vi "4Pi Dual DM - Mode Scan Engine.vi"() -> ()   [LabVIEW 2016]
uses:
  4Pi Dual DM - Controls/4Pi Dual DM - Mode Scan - Gaussian Initial Guesses.ctl
  4Pi Dual DM - Controls/4Pi Dual DM - Mode Scan - Metric Fit Type.ctl
  4Pi Dual DM - Controls/4Pi Dual DM - Mode Scan - Scan Settings.ctl
  4Pi Dual DM - Controls/4Pi Dual DM - Mode Scan - Metric.ctl
  4Pi Dual DM - Controls/4Pi Dual DM - Mode Scan - Threshold Mean Limits.ctl
  4Pi Dual DM - Controls/4Pi Dual DM - Mode Scan - Image Type.ctl
  4Pi Dual DM - Controls/4Pi Dual DM - Mode Scan - Blink Scan Settings.ctl
  4Pi Dual DM - Controls/4Pi Dual DM - Mode Scan - Blink Analysis Type.ctl
  <vilib>/vision/Image Controls.llb/IMAQ Image.ctl
  Hardware Configuration/Hardware Configuration Controls/Device Type.ctl
  Hardware Configuration/Hardware Configuration Controls/Device Function.ctl
  <vilib>/Utility/miscctls.llb/LVPointTypeDef.ctl
  4Pi Dual DM - Controls/4Pi Dual DM - Mode Scan - Last Used Data Type.ctl
  4Pi Dual DM - Controls/4Pi Dual DM - Mode Scan - Notifier Type.ctl
  4Pi Dual DM - Controls/4Pi Dual DM - Mode Scan - Scan Actions.ctl
  4Pi Dual DM - Controls/4Pi Dual DM - Standard Action.ctl
  4Pi Dual DM - Controls/4Pi Dual DM - Standard Counter Action.ctl
  <vilib>/Analysis/6fits.llb/Curve Fitting Criteria.ctl
  <vilib>/Analysis/baseanly.llb/Mean (DBL).vi
  <vilib>/Analysis/NI_AALBase.lvlib
  <vilib>/Analysis/NI_AALPro.lvlib
  <vilib>/gmath/NI_Gmath.lvlib
  <resource>/objmgr/IMAQImage.rc
panel:
  in  "Current Mode":i32(ring) items=["1", "2", "3", "4", "5", "6", "7", "8", "9", "10", "11", "12", "13", "14", "15", "16", "17", "18", "19", "20", "21", "22", "23", "24", "25", "26", "27", "28", "29", "30", "31", "32", "33", "34", "35", "36", "37", "38", "39", "40", "41", "42", "43", "44", "45", "46", "47", "48", "49", "50", "51", "52", "53", "54", "55", "56", "57", "58", "59", "60", "61", "62", "63", "64", "65", "66", "67", "68", "69", "70", "71", "72", "73", "74", "75", "76", "77", "78", "79", "80", "81", "82", "83", "84", "85", "86", "87", "88", "89", "90", "91", "92", "93", "94", "95", "96", "97", "98", "99", "100", "101", "102", "103", "104", "105", "106", "107", "108", "109", "110", "111", "112", "113", "114", "115", "116", "117", "118", "119", "120", "121", "122", "123", "124", "125", "126", "127", "128", "129", "130", "131", "132", "133", "134", "135", "136", "137", "138", "139", "140"]
  in  "Scan Mode":bool
  in  "Scan Next Mode":bool
  in  "Auto Scan Modes":bool
  in  "Calling VI Ref":refnum<vi>
  in  "Main Tab":enum32{"Scan Modes", "Settings"}(tab)
  in  "Blink Scan Settings":T1={"Blink Analysis Type"=1, "Blink ROI Box Width"=0, "Blink Threshold"=0.0} {"Blink Analysis Type" items=["Mean Intensity", "2D Fit Intensity"]}
  in  "Fit Data":bool
  in  "Apply":bool
  in  "Get Image":bool
  in  "Image Type":T3 items=["Full Image", "ROI", "Blinks"]
  in  "Fit Type":T4 items=["Guassian", "Quadratic"]
  in  "Gaussian Initial Guesses":T5={"Amplitude"=2500.0, "Center Position"=0.0, "Width (Sigma)"=200.0, "Offset"=500.0, "User Guesses"=TRUE}
  in  "DM Scan Settings":T6={"Frame Delay"=1, "Frame Accumulations"=2, "Number of Steps"=8, "Step Size (nm)"=80}
  in  "Metric":T7=1 items=["Max Intensity", "No Zero Mean", "Threshold Mean", "Mean"]
  in  "Image Selection":i32(ring) items=["Quad 01", "Quad 02", "Quad 03", "Quad 04"]
  in  "Threshold Mean Limits":T8={"Upper Limit"=10000.0, "Lower Limit"=0.0}
  out "Metric":cluster{dbl[], dbl[]}[](graph)
  out "Image":u16[][](graph)
  in  "Exit":bool
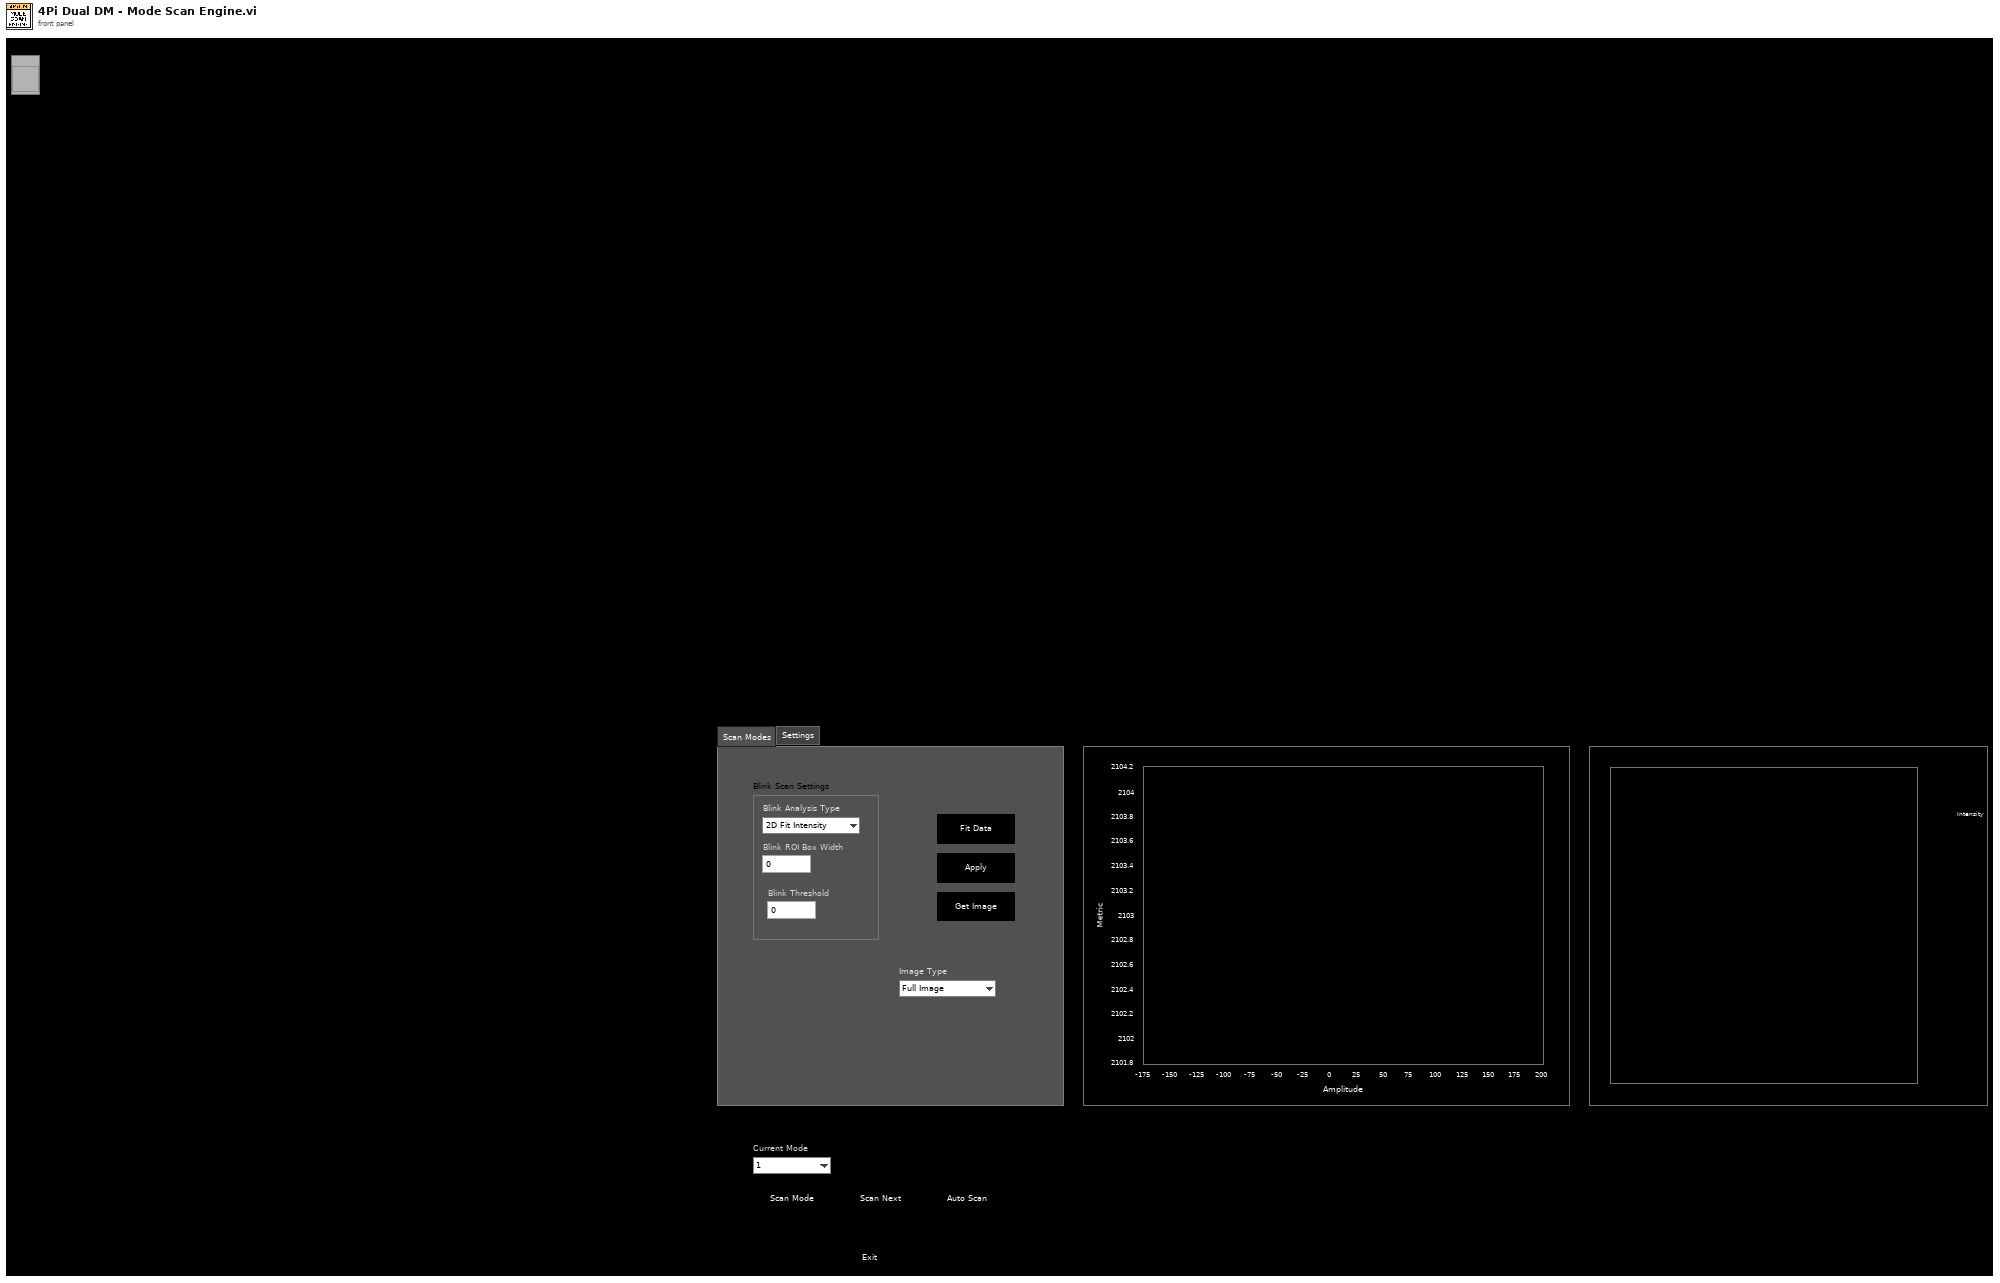
[diagram p1: front panel]
types:
  T1 = typedef "4Pi Dual DM - Mode Scan - Blink Scan Settings.ctl" = cluster{"Blink Analysis Type":T2, "Blink ROI Box Width":u8, "Blink Threshold":dbl}
  T2 = typedef "4Pi Dual DM - Mode Scan - Blink Analysis Type.ctl" = u16
  T3 = typedef "4Pi Dual DM - Mode Scan - Image Type.ctl" = u16
  T4 = typedef "4Pi Dual DM - Mode Scan - Metric Fit Type.ctl" = u16
  T5 = typedef "4Pi Dual DM - Mode Scan - Gaussian Initial Guesses.ctl" = cluster{"Amplitude":dbl, "Center Position":dbl, "Width (Sigma)":dbl, "Offset":dbl, "User Guesses":bool}
  T6 = typedef "4Pi Dual DM - Mode Scan - Scan Settings.ctl" = cluster{"Frame Delay":u32, "Frame Accumulations":u16, "Number of Steps":u16, "Step Size (nm)":u16}
  T7 = typedef "4Pi Dual DM - Mode Scan - Metric.ctl" = u16
  T8 = typedef "4Pi Dual DM - Mode Scan - Threshold Mean Limits.ctl" = cluster{"Upper Limit":dbl, "Lower Limit":dbl}
  T9 = typedef "4Pi Dual DM - Mode Scan - Scan Actions.ctl" = enum16{"Scan Mode", "Fit Data", "Scan Next Mode", "Update Mode Amount", "Get Image", "Compute Metric", "Update Counter", "Apply Correction", "Exit", "Quit"}
  T10 = typedef "4Pi Dual DM - Mode Scan - Notifier Type.ctl" = cluster{"Action":T9, "Image Ref":T11, "Image Type":T3, "Fit Type":T4, "Metric":T7, "Scan Running?":bool, "DM Scan Settings":T6, "Threshold Mean Limits":T8, "Gaussian Initial Guesses":T5, "Blink Scan Settings":T1}
  T11 = typedef "IMAQ Image.ctl" = refnum<image>
  T12 = typedef "4Pi Dual DM - Mode Scan - Last Used Data Type.ctl" = cluster{"Image Ref Index":i32, "Image Type":T3, "Fit Type":T4, "Metric":T7, "DM Scan Settings":T6, "Threshold Mean Limits":T8, "Gaussian Initial Guesses":T5, "Blink Scan Settings":T1}
  T13 = enum16{"Always On", "Always Off", "Off While Running"}
  T14 = typedef "LVPointTypeDef.ctl" = cluster{"Horizontal":i16, "Vertical":i16}
  T15 = typedef "Device Function.ctl" = enum16{"Primary", "Secondary", "Overview", "Wide Field Drift Correction", "642 nm Excitation", "560 nm Excitation", "546 nm Excitation", "488 nm Excitation", "405 nm Excitation", "Objective Drift Correction", "Objective XY", "Objective Z", "Sample XY", "Sample Coarse Z", "Sample Z", "4Pi Lower", "4Pi Upper", "Adj Cavity", "Line Scanning"}
  T16 = typedef "Device Type.ctl" = enum16{"AOTF", "Camera", "Deformable Mirror", "Laser", "Shutter", "Stage", "Waveform"}
  T17 = typedef "LVRectTypeDef.ctl" = cluster{"Left":i16, "Top":i16, "Right":i16, "Bottom":i16}
  T18 = typedef "LVBoundsTypeDef.ctl" = cluster{"Width":u32, "Height":u32}
  T19 = typedef "4Pi Dual DM - Standard Action.ctl" = enum16{"Read", "Write"}
  T20 = typedef "4Pi Dual DM - Standard Counter Action.ctl" = enum16{"Initialize", "Update Count", "Get Count"}
  T21 = cluster{"initial amplitude":dbl, "initial center":dbl, "initial standard deviation":dbl, "offset":dbl}
  T22 = cluster{"amp min":dbl, "amp max":dbl, "center min":dbl, "center max":dbl, "deviation min":dbl, "deviation max":dbl, "offset min":dbl, "offset max":dbl}
  T23 = enum16{"Linear", "Polynomial", "Exponential", "Power"}
  T24 = enum8{"Enabled", "Disabled", "Disabled and Grayed Out"}
  T25 = typedef "4Pi Dual DM - Mirror Modes DUAL.ctl" = cluster{"Mode":string, "Amplitude":dbl}[][]
  T26 = cluster{"Amplitude Out":dbl[], "Metric Out":dbl[]}
  T27 = cluster{"initial amplitude":dbl, "Numeric":dbl, "initial standard deviation":dbl, "offset":dbl}
  T28 = typedef "NI_AALPro.lvlib/Curve Fitting Criteria.ctl" = u16
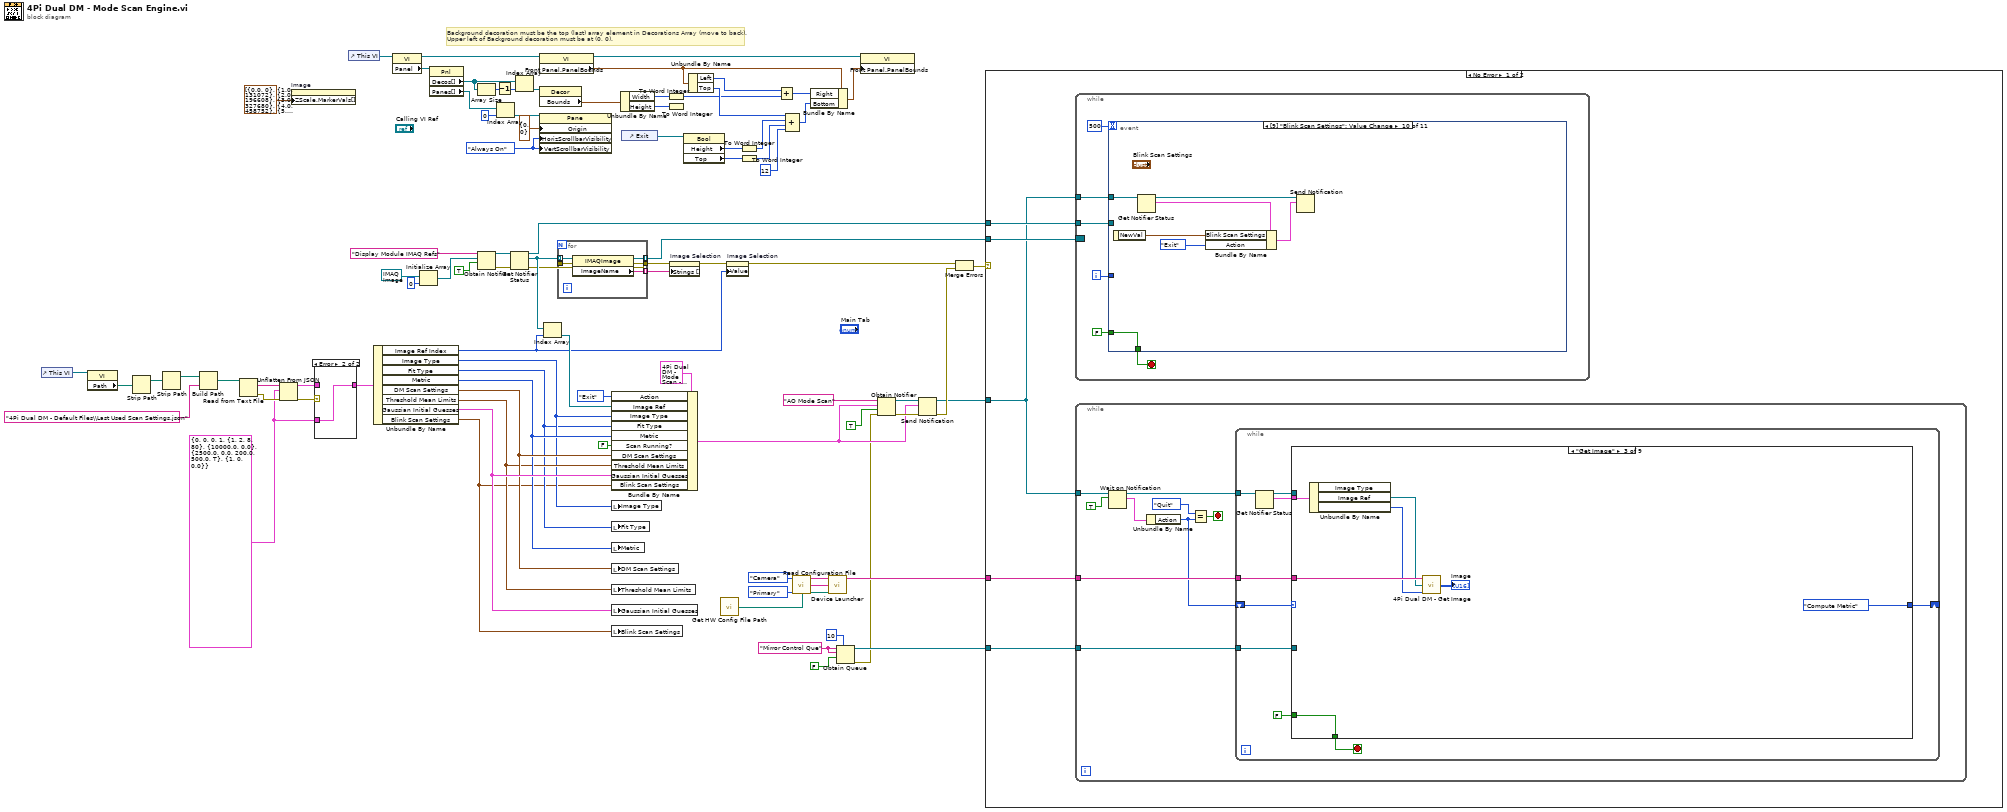
[diagram p0: block diagram]
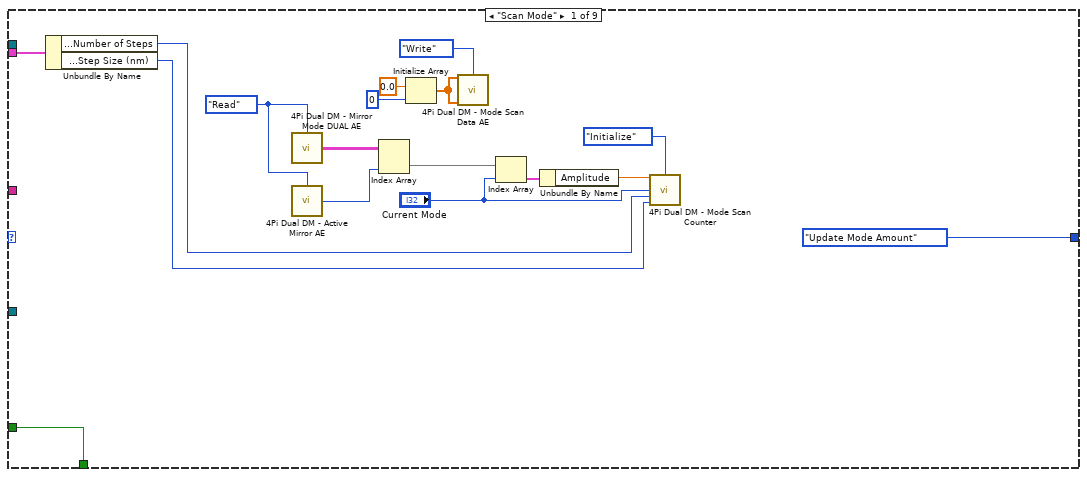
[diagram p2: hidden frame]
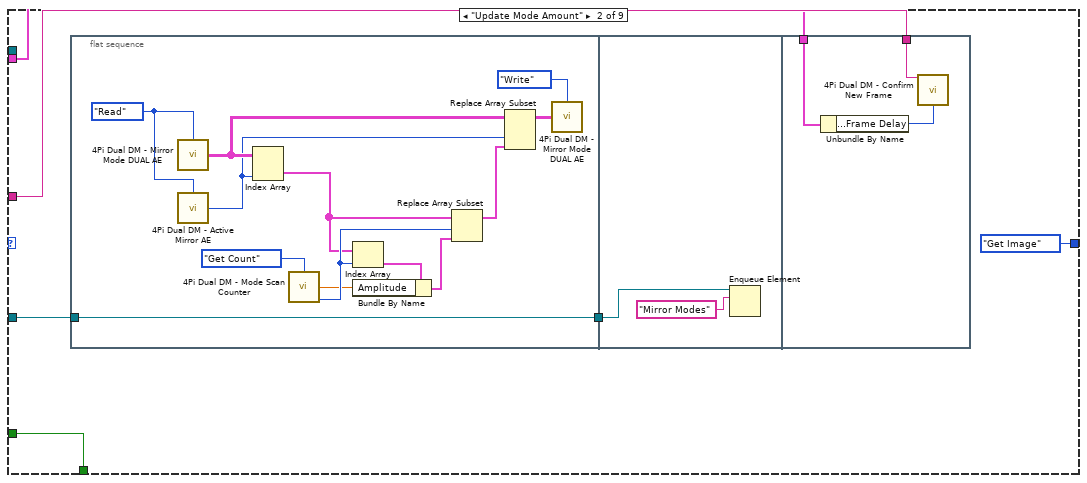
[diagram p3: hidden frame]
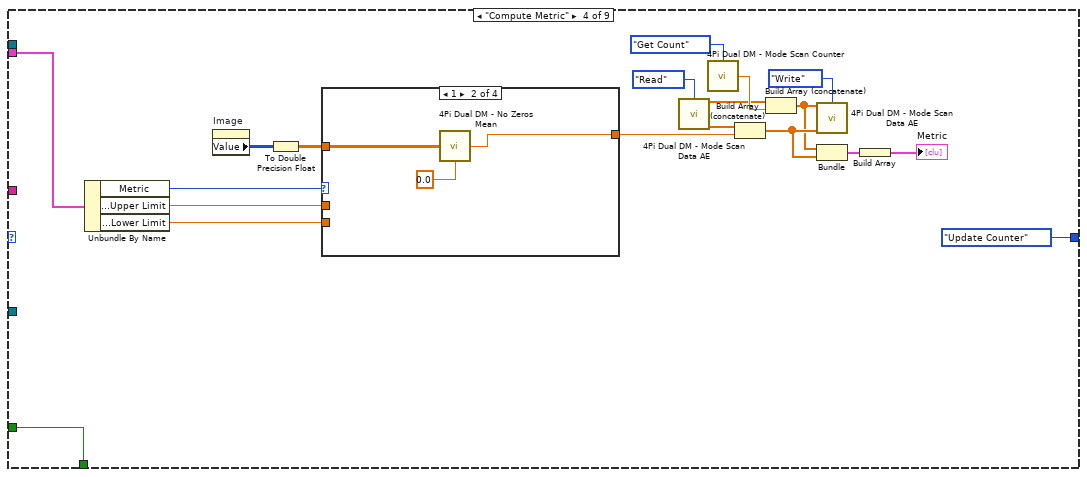
[diagram p4: hidden frame]
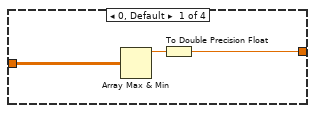
[diagram p5: hidden frame]
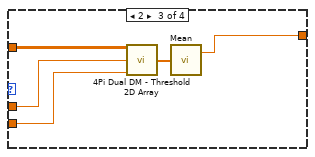
[diagram p6: hidden frame]
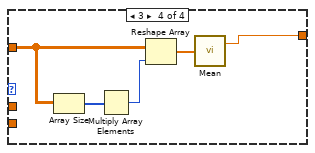
[diagram p7: hidden frame]
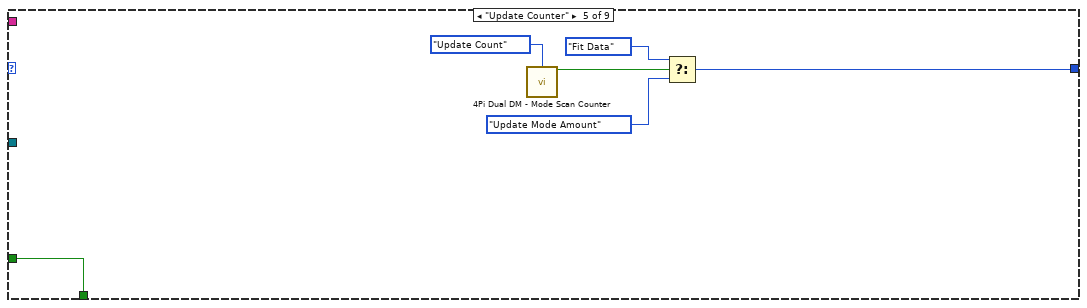
[diagram p8: hidden frame]
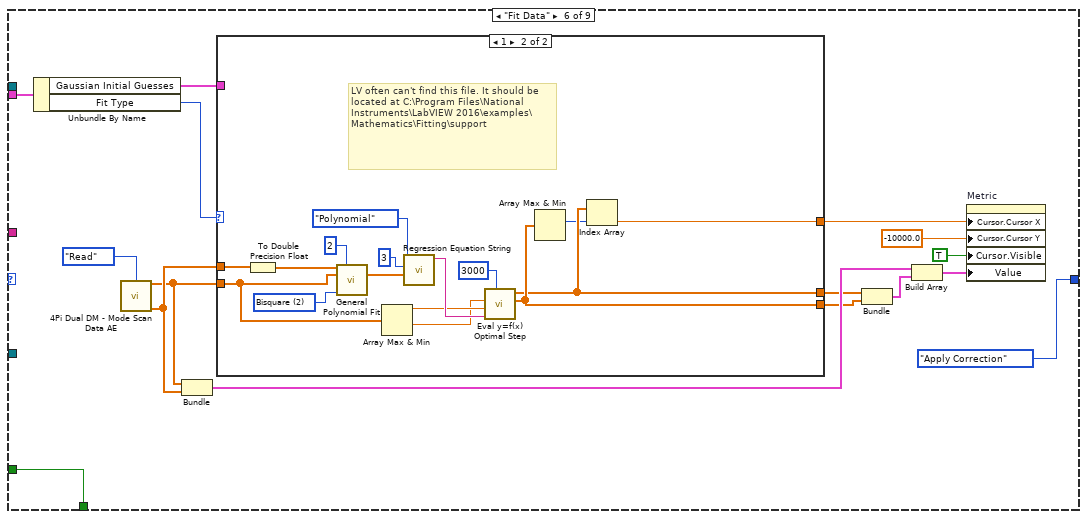
[diagram p9: hidden frame]
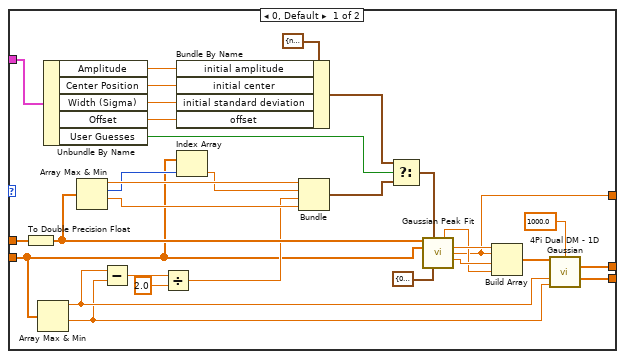
[diagram p10: hidden frame]
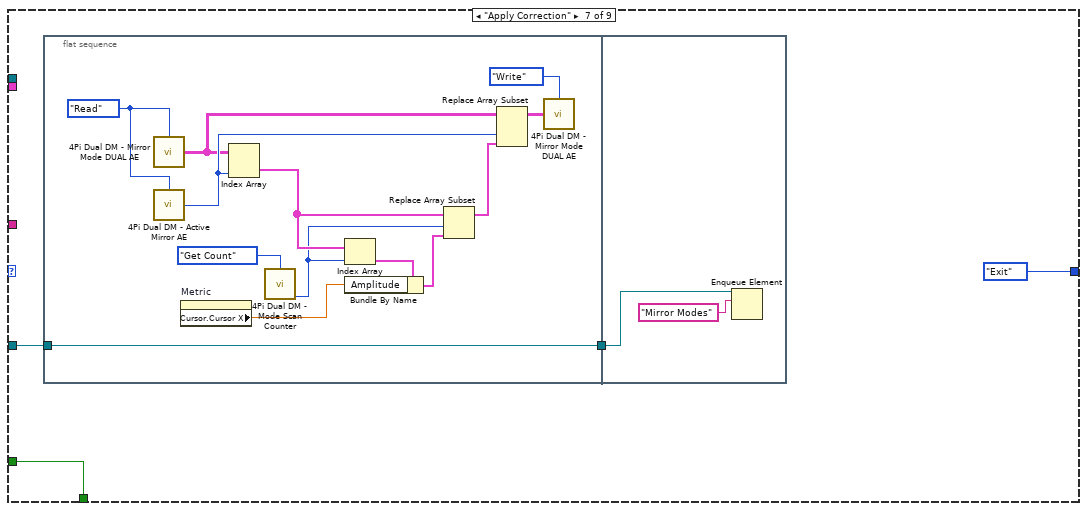
[diagram p11: hidden frame]
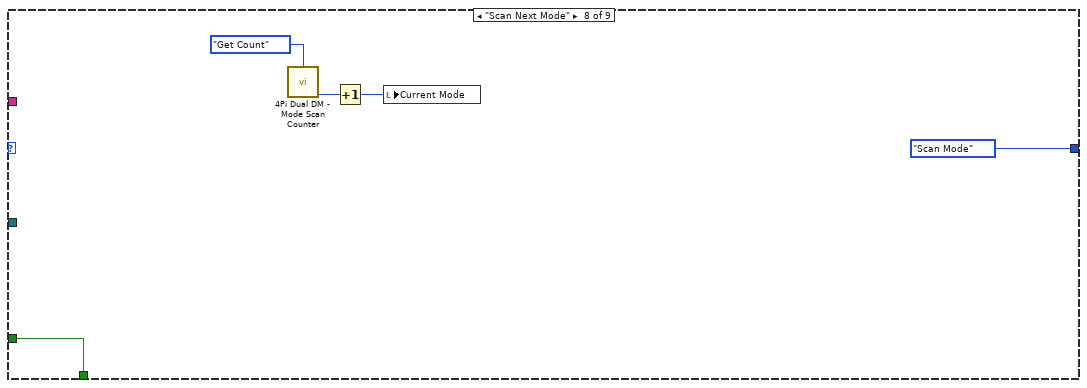
[diagram p12: hidden frame]
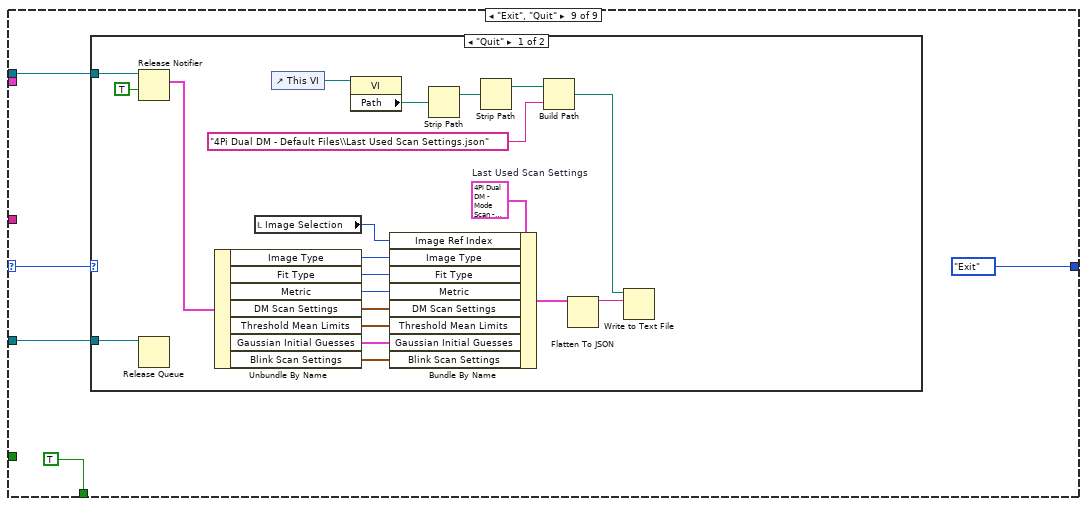
[diagram p13: hidden frame]
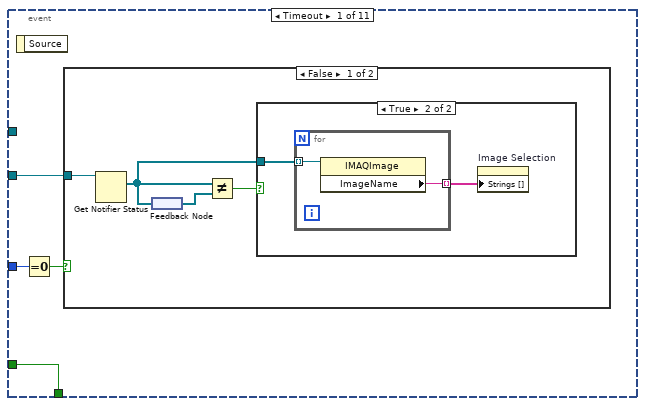
[diagram p15: hidden frame]
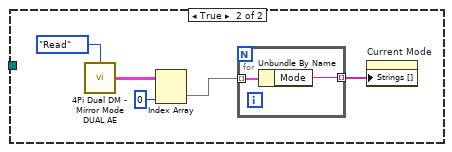
[diagram p17: hidden frame]
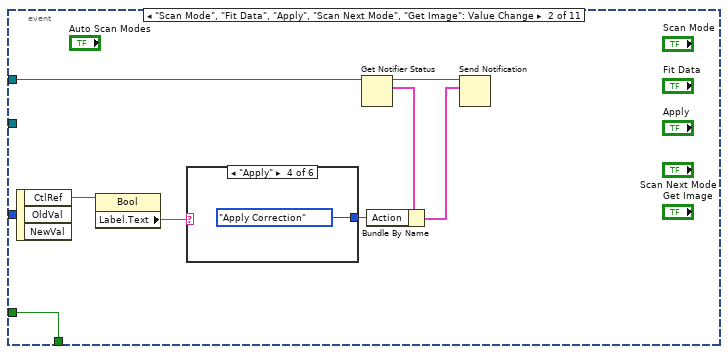
[diagram p18: hidden frame]
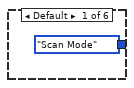
[diagram p19: hidden frame]
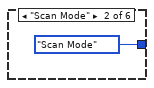
[diagram p20: hidden frame]
diagram:
  w24 = T12 {"Image Ref Index"=0, "Image Type"=0, "Fit Type"=0, "Metric"=1, "DM Scan Settings"={"Frame Delay"=1, "Frame Accumulations"=2, "Number of Steps"=8, "Step Size (nm)"=80}, "Threshold Mean Limits"={"Upper Limit"=10000.0, "Lower Limit"=0.0}, "Gaussian Initial Guesses"={"Amplitude"=2500.0, "Center Position"=0.0, "Width (Sigma)"=200.0, "Offset"=500.0, "User Guesses"=TRUE}, "Blink Scan Settings"={"Blink Analysis Type"=1, "Blink ROI Box Width"=0, "Blink Threshold"=0.0}} ("Mode Scan Notifier Type")
  w55 = T13."Always On" ("Vertical Scrollbar Visibility")
  w89 = "Mirror Control Que" ("name (unnamed)")
  # "Background decoration must be the top (last) array element in Decorations Array (move to back).\nUpper left of Background decoration must be at (0, 0)."
  n1 = control-ref of="This VI"() -> (w37:refnum<vi>)
  n2 = property class="VI"(reference=w37) -> ("Path"=w36:path)  [unwired: 1 in, 2 out]
  n3 = Strip Path(path=w36) -> (stripped path=w35:path)  [unwired: 1 out]
  n4 = Strip Path(path=w35) -> (stripped path=w34:path)  [unwired: 1 out]
  n5 = Build Path(base path=w34, name or relative path="4Pi Dual DM - Default Files\\Last Used Scan Settings.json") -> (appended path=w31:path)
  n6 = Read from Text File(file (use dialog)=w31) -> (text=w32:string, error out=w30:errorcluster)  [unwired: 3 in, 2 out]
  n7 = Unflatten From JSON(JSON string=w32, type and defaults=w24, error in (no error)=w30) -> (value=w23:T12, error out=w29:errorcluster)  [unwired: 4 in]
  n8 = property on="Image" class="IntGraph (strict)"("ZScale.MarkerVals[]"=cluster{dbl, u32}[] [{0.0, 0}, {1.0, 131072}, {2.0, 196608}, {3.0, 327680}, {4.0, 458752}, {5.0, 589824}, {6.0, 720896}, {7.0, 851971}, {8.0, 983043}, {9.0, 1114115}, {10.0, 1245187}, {11.0, 1376259}, {12.0, 1507331}, {13.0, 1638403}, {14.0, 1769475}, {15.0, 1769479}, {16.0, 2031623}, {17.0, 2162695}, {18.0, 2293767}, {19.0, 2424839}, {20.0, 2555911}, {21.0, 2686983}, {22.0, 2818055}, {23.0, 2949127}, {24.0, 3080203}, {25.0, 3211275}, {26.0, 3342347}, {27.0, 3473419}, {28.0, 3604491}, {29.0, 3735563}, {30.0, 3866635}, {31.0, 3867403}, {32.0, 4129547}, {33.0, 4260619}, {34.0, 4391691}, {35.0, 4522763}, {36.0, 4653839}, {37.0, 4784911}, {38.0, 4915983}, {39.0, 5178127}, {40.0, 5309199}, {41.0, 5440271}, {42.0, 5571343}, {43.0, 5702415}, {44.0, 5703439}, {45.0, 5965583}, {46.0, 6096655}, {47.0, 6227727}, {48.0, 6358799}, {49.0, 6489871}, {50.0, 6620943}, {51.0, 6752015}, {52.0, 6883087}, {53.0, 7015183}, {54.0, 7146255}, {55.0, 7277327}, {56.0, 7408399}, {57.0, 7539471}, {58.0, 7670543}, {59.0, 7801615}, {60.0, 8063759}, {61.0, 8194831}, {62.0, 8326927}, {63.0, 8457999}, {64.0, 8589075}, {65.0, 8720147}, {66.0, 8851219}, {67.0, 8982291}, {68.0, 9113363}, {69.0, 9114387}, {70.0, 9376531}, {71.0, 9507603}, {72.0, 9638675}, {73.0, 9769747}, {74.0, 9901843}, {75.0, 10032915}, {76.0, 10163987}, {77.0, 10229523}, {78.0, 10295059}, {79.0, 10427155}, {80.0, 10558227}, {81.0, 10689299}, {82.0, 10820371}, {83.0, 10886931}, {84.0, 10952467}, {85.0, 11083539}, {86.0, 11214611}, {87.0, 11215635}, {88.0, 11477779}, {89.0, 11543315}, {90.0, 11608851}, {91.0, 11740947}, {92.0, 11806483}, {93.0, 11872019}, {94.0, 12004115}, {95.0, 12135187}, {96.0, 12266259}, {97.0, 12267283}, {98.0, 12398355}, {99.0, 12529427}, {100.0, 12530451}, {101.0, 12595987}, {102.0, 12530451}, {103.0, 12793619}, {104.0, 12794131}, {105.0, 12794643}, {106.0, 13056787}, {107.0, 13057299}, {108.0, 13057811}, {109.0, 13188883}, {110.0, 13320979}, {111.0, 13386515}, {112.0, 13452563}, {113.0, 13584147}, {114.0, 13584659}, {115.0, 13585171}, {116.0, 13585683}, {117.0, 13717267}, {118.0, 13848339}, {119.0, 13849363}, {120.0, 13849875}, {121.0, 13850387}, {122.0, 13981459}, {123.0, 14113555}, {124.0, 14114067}, {125.0, 14114579}, {126.0, 14115091}, {127.0, 14246675}, {128.0, 14377747}, {129.0, 14378771}, {130.0, 14379283}, {131.0, 14379539}, {132.0, 14379795}, {133.0, 14380819}, {134.0, 14511891}, {135.0, 14643987}, {136.0, 14644503}, {137.0, 14645015}, {138.0, 14645527}, {139.0, 14646039}, {140.0, 14646551}, {141.0, 14778135}, {142.0, 14909207}, {143.0, 14910231}, {144.0, 14910747}, {145.0, 14911259}, {146.0, 14911771}, {147.0, 14912283}, {148.0, 14912797}, {149.0, 15044383}, {150.0, 15175455}, {151.0, 15175967}, {152.0, 15176479}, {153.0, 15176991}, {154.0, 15177507}, {155.0, 15178019}, {156.0, 15178531}, {157.0, 15310115}, {158.0, 15441701}, {159.0, 15441959}, {160.0, 15442215}, {161.0, 15442727}, {162.0, 15443243}, {163.0, 15443755}, {164.0, 15444269}, {165.0, 15444783}, {166.0, 15444783}, {167.0, 15576367}, {168.0, 15707953}, {169.0, 15708467}, {170.0, 15708979}, {171.0, 15708981}, {172.0, 15708983}, {173.0, 15710011}, {174.0, 15710523}, {175.0, 15711037}, {176.0, 15711039}, {177.0, 15711553}, {178.0, 15843139}, {179.0, 15974213}, {180.0, 15974215}, {181.0, 15974217}, {182.0, 15974219}, {183.0, 15975755}, {184.0, 15976271}, {185.0, 15976785}, {186.0, 15977299}, {187.0, 15977301}, {188.0, 15977815}, {189.0, 15978327}, {190.0, 15978331}, {191.0, 16109917}, {192.0, 16241503}, {193.0, 16241505}, {194.0, 16242019}, {195.0, 16242535}, {196.0, 16242537}, {197.0, 16242539}, {198.0, 16243563}, {199.0, 16243567}, {200.0, 16244081}, {201.0, 16244595}, {202.0, 16244599}, {203.0, 16244601}, {204.0, 16244603}, {205.0, 16245627}, {206.0, 16245631}, {207.0, 16245633}, {208.0, 16246147}, {209.0, 16246663}, {210.0, 16377735}, {211.0, 16508811}, {212.0, 16508815}, {213.0, 16509839}, {214.0, 16509843}, {215.0, 16509845}, {216.0, 16509847}, {217.0, 16510361}, {218.0, 16510875}, {219.0, 16510879}, {220.0, 16510881}, {221.0, 16510883}, {222.0, 16511399}, {223.0, 16511911}, {224.0, 16511915}, {225.0, 16511917}, {226.0, 16511919}, {227.0, 16511923}, {228.0, 16512437}, {229.0, 16512951}, {230.0, 16512955}, {231.0, 16512957}, {232.0, 16512959}, {233.0, 16512961}, {234.0, 16512963}, {235.0, 16512967}, {236.0, 16513481}, {237.0, 16513995}, {238.0, 16513999}, {239.0, 16514001}, {240.0, 16514003}, {241.0, 16514005}, {242.0, 16514007}, {243.0, 16514011}, {244.0, 16514013}, {245.0, 16514015}, {246.0, 16514019}, {247.0, 16514021}, {248.0, 16514023}, {249.0, 16514027}, {250.0, 16514029}, {251.0, 16514031}, {252.0, 16514035}, {253.0, 16514037}, {254.0, 16514039}, {255.0, 16514043}] ("Z Scale.Marker Values[]")) -> ()  [unwired: 2 in, 2 out]
  n9 = case shown="Error" w29 {
    tunnel: w24 -> [_ w91]
    tunnel: w23 -> [w90 _]
    tunnel: [w90 w91] -> w20
    frame No Error {
    }
    frame Error {
    }
  }
  n10 = control-ref of="This VI"() -> (w47:refnum<vi>)
  n11 = Unbundle By Name(w20) -> ("Image Ref Index"=w18:i32, "Image Type"=w3:T3, "Fit Type"=w2:T4, "Metric"=w5:T7, "DM Scan Settings"=w6:T6, "Threshold Mean Limits"=w4:T8, "Gaussian Initial Guesses"=w7:T5, "Blink Scan Settings"=w1:T1)
  n12 = property class="VI"(reference=w47) -> (reference out=w56:refnum<vi>, "Panel"=w48:refnum<vi>)  [unwired: 1 in, 1 out]
  n13 = Initialize Array(T11 refnum ("New Image"), 0 ("dimension size")) -> (w81:T11[])
  n14 = property class="Pnl"(reference=w48) -> ("Decos[]"=w46:refnum<vi>[], "Panes[]"=w52:refnum<vi>[])  [unwired: 1 in, 2 out]
  n15 = Obtain Notifier(name (unnamed)="Display Module IMAQ Refs", notification data type=w81, create if not found? (T)=TRUE) -> (notifier out=w80:refnum<notifier>, error out=w42:errorcluster)  [unwired: 1 in, 1 out]
  n16 = Array Size(array=w46) -> (size(s)=w44:i32)
  n17 = Decrement(x=w44) -> (x-1=w45:i32)
  n18 = Index Array(array=w52, index=0) -> (element=w51:refnum<vi>)
  n19 = Get Notifier Status(notifier=w80, error in (no error)=w42) -> (notifier out=w13:refnum<notifier>, current notification=w43:T11[], error out=w41:errorcluster)  [unwired: 2 out]
  n20 = Index Array(array=w46, index=w45) -> (element=w54:refnum<vi>)
  n21 = property class="VI"(reference=w56) -> (reference out=w58:refnum<vi>, "Front Panel.PanelBounds"=w59:T17)  [unwired: 1 in, 1 out]
  n22 = property class="Decor"(reference=w54) -> ("Bounds"=w57:T18)  [unwired: 1 in, 2 out]
  n23 = property class="Pane"(reference=w51, "Origin"=T14 {"Horizontal"=0, "Vertical"=0}, "HorizScrollbarVisibility"=w55, "VertScrollbarVisibility"=w55) -> ()  [unwired: 1 in, 2 out]
  n24 = Index Array(array=w43, index=w18) -> (element=w19:T11)
  n25 = for {
    tunnel: w43 -> [w96] mode=indexing
    tunnel: [w95] -> w40 mode=indexing
    tunnel: [w94] -> w39
    tunnel: [w93] -> w12 mode=indexing
    tunnel: w41 -> [w92]
    n26 = property class="IMAQImage"(reference=w96, error in=w92) -> (reference out=w93:T11, error out=w94:errorcluster, "ImageName"=w95:string)
  }
  n27 = Bundle By Name(cluster=T10 {"Action"=enum."Scan Mode", "Image Ref"=refnum, "Image Type"=0, "Fit Type"=0, "Metric"=1, "Scan Running?"=FALSE, "DM Scan Settings"={"Frame Delay"=1, "Frame Accumulations"=2, "Number of Steps"=8, "Step Size (nm)"=80}, "Threshold Mean Limits"={"Upper Limit"=10000.0, "Lower Limit"=0.0}, "Gaussian Initial Guesses"={"Amplitude"=2500.0, "Center Position"=0.0, "Width (Sigma)"=200.0, "Offset"=500.0, "User Guesses"=TRUE}, "Blink Scan Settings"={"Blink Analysis Type"=1, "Blink ROI Box Width"=0, "Blink Threshold"=0.0}} ("Mode Scan Notifier Type"), "Action"=4Pi_Dual_DM_-_Mode_Scan_-_Scan_Actions."Exit", "Image Ref"=w19, "Image Type"=w3, "Fit Type"=w2, "Metric"=w5, "Scan Running?"=FALSE, "DM Scan Settings"=w6, "Threshold Mean Limits"=w4, "Gaussian Initial Guesses"=w7, "Blink Scan Settings"=w1) -> (w16:T10)
  n28 = local write "Image Type"(w3) -> ()
  n29 = local write "Fit Type"(w2) -> ()
  n30 = local write "Metric"(w5) -> ()
  n31 = local write "DM Scan Settings"(w6) -> ()
  n32 = local write "Threshold Mean Limits"(w4) -> ()
  n33 = local write "Gaussian Initial Guesses"(w7) -> ()
  n34 = local write "Blink Scan Settings"(w1) -> ()
  n35 = Unbundle By Name(w57) -> ("Width"=w62:u32, "Height"=w65:u32)
  n36 = control-ref of="Exit"() -> (w49:refnum<vi>)
  n37 = To Word Integer(number=w62) -> (16bit integer=w64:i16)
  n38 = To Word Integer(number=w65) -> ()  [unwired: 1 out]
  n39 = property on="Image Selection" class="Ring (strict)"(error in=w39, "Strings []"=w40) -> (error out=w38:errorcluster)  [unwired: 1 in, 1 out]
  n40 = property class="Bool"(reference=w49) -> ("Height"=w67:u32, "Top"=w68:i32)  [unwired: 1 in, 2 out]
  n41 = Unbundle By Name(w59) -> ("Left"=w61:i16, "Top"=w72:i16)
  n42 = call "Get HW Config File Path.vi"() -> ("File Path"=w74:path)  [unwired: 14 in, 1 out]
  n43 = property on="Image Selection" class="Ring (strict)"(error in=w38, "Value"=w18) -> (error out=w11:errorcluster)  [unwired: 1 in, 1 out]
  n44 = To Word Integer(number=w67) -> (16bit integer=w70:i16)
  n45 = To Word Integer(number=w68) -> (16bit integer=w71:i16)
  n46 = Add(x=w61, y=w64) -> (x+y=w63:i16)
  n47 = Compound Arithmetic op=ADD(w72, w70, w71, i16 12 ("y")) -> (w66:i16)
  n48 = call "Read Configuration File.vi"("Device Type"=Device_Type."Camera", "Device Function"=Device_Function."Primary", "Config File Path"=w74) -> ("Unique Notifier Name"=w75:string, "Device Ports/IDs/Channels"=w77:string[], "Device Engine Path"=w76:path)  [unwired: 9 in, 1 out]
  n49 = Bundle By Name(cluster=w59, "Right"=w63, "Bottom"=w66) -> (w60:T17)
  n50 = call "Device Launcher.vi"("Notifier Name"=w75, "Device Ports/IDs/Channels"=w77, "Device Engine Path"=w76) -> ("Notifier Name"=w73:string)  [unwired: 11 in, 1 out]
  n51 = Obtain Queue(max queue size (-1, unlimited)=10, name (unnamed)=w89, element data type=w89, create if not found? (T)=FALSE) -> (queue out=w87:refnum<queue>, error out=w14:errorcluster)  [unwired: 1 in, 1 out]
  n52 = property class="VI"(reference=w58, "Front Panel.PanelBounds"=w60) -> ()  [unwired: 1 in, 2 out]
  n53 = Obtain Notifier(name (unnamed)="AO Mode Scan", notification data type=w16, create if not found? (T)=TRUE, error in (no error)=w14) -> (notifier out=w25:refnum<notifier>, error out=w26:errorcluster)  [unwired: 1 out]
  n54 = Send Notification(notification=w16, notifier=w25, error in (no error)=w26) -> (notifier out=w8:refnum<notifier>, error out=w10:errorcluster)
  n55 = Merge Errors(w11, w10) -> (w9:errorcluster)
  n56 = case shown="No Error" w9 {
    tunnel: w87 -> [w101 _]
    tunnel: w73 -> [w100 _]
    tunnel: w13 -> [w99 _]
    tunnel: w12 -> [w98 _]
    tunnel: w8 -> [w97 _]
    frame No Error {
      n57 = while {
        tunnel: w99 -> [w325]
        border: w98 -> [_]
        tunnel: w97 -> [w324]
        i -> [w327]
        stop <- w322 stop-if-true
        n58 = event shown="[9] \"Blink Scan Settings\": Value Change" {
          selector: _ -> [_ _ _ _ _ _ _ _ _ _ _]
          dyn-events: _ -> [_ _ _ _ _ _ _ _ _ _ _]
          timeout: 500 -> [_ _ _ _ _ _ _ _ _ _ _]
          tunnel: w327 -> [w331 _ _ _ _ _ _ _ _ _ _]
          tunnel: w325 -> [w329 _ w370 _ _ _ _ _ _ _ w429]
          tunnel: w324 -> [_ w353 w369 w378 w386 w393 w401 w408 w415 w422 w427]
          tunnel: [w328 w347 w361 w371 w387 w394 w395 w402 w409 w416 TRUE] -> w322
          tunnel: FALSE -> [w328 w347 w361 w371 w387 w394 w395 w402 w409 w416 _]
          event Timeout {
            n59 = event-data() -> ()  [unwired: 1 in, 1 out]
            n60 = Equal To 0?(x=w331) -> (x = 0?=w330:bool)
            n61 = case shown="False" w330 {
              tunnel: w329 -> [w335 _]
              frame False {
                n62 = Get Notifier Status(notifier=w335) -> (current notification=w332:T11[])  [unwired: 1 in, 4 out]
                n63 = feedback-in #1(w332) -> ()
                n64 = feedback #1() -> (w334:T11[])
                n65 = Not Equal?(x=w332, y=w334) -> (x != y?=w333:bool)
                n66 = case shown="True" w333 {
                  tunnel: w332 -> [_ w337]
                  frame False {
                  }
                  frame True {
                    n67 = for {
                      tunnel: w337 -> [w339] mode=indexing
                      tunnel: [w338] -> w336 mode=indexing
                      n68 = property class="IMAQImage"(reference=w339) -> ("ImageName"=w338:string)  [unwired: 1 in, 2 out]
                    }
                    n69 = property on="Image Selection" class="Ring (strict)"("Strings []"=w336) -> ()  [unwired: 2 in, 2 out]
                  }
                }
              }
              frame True {
                n70 = call "4Pi Dual DM - Mirror Mode DUAL AE.vi"("Action"=4Pi_Dual_DM_-_Standard_Action."Read") -> ("Mirror Modes Out"=w342:T25)  [unwired: 14 in]
                n71 = Index Array(array=w342, index (col)=0 ("disabled index (col)")) -> (element=w340:cluster{"Mode":string, "Amplitude":dbl}[])  [unwired: 1 in]
                n72 = for {
                  tunnel: w340 -> [w346] mode=indexing
                  tunnel: [w345] -> w344 mode=indexing
                  n73 = Unbundle By Name(w346) -> ("Mode"=w345:string)
                }
                n74 = property on="Current Mode" class="Ring (strict)"("Strings []"=w344) -> ()  [unwired: 2 in, 2 out]
              }
            }
          }
          event "Scan Mode", "Fit Data", "Apply", "Scan Next Mode", "Get Image": Value Change {
            n75 = event-data() -> ("CtlRef"=w354:refnum<vi>)  [unwired: 1 in, 2 out]
            n76 = property class="Bool"(reference=w354) -> ("Label.Text"=w349:string)  [unwired: 1 in, 2 out]
            n77 = case shown="\"Apply\"" w349 {
              tunnel: [4Pi_Dual_DM_-_Mode_Scan_-_Scan_Actions."Scan Mode" ("Action") 4Pi_Dual_DM_-_Mode_Scan_-_Scan_Actions."Scan Mode" ("Action") 4Pi_Dual_DM_-_Mode_Scan_-_Scan_Actions."Fit Data" ("Action") 4Pi_Dual_DM_-_Mode_Scan_-_Scan_Actions."Apply Correction" ("Action") 4Pi_Dual_DM_-_Mode_Scan_-_Scan_Actions."Scan Next Mode" ("Action") 4Pi_Dual_DM_-_Mode_Scan_-_Scan_Actions."Get Image" ("Action")] -> w348
              frame Default {
              }
              frame "Scan Mode" {
              }
              frame "Fit Data" {
              }
              frame "Apply" {
              }
              frame "Scan Next Mode" {
              }
              frame "Get Image" {
              }
            }
            n78 = Get Notifier Status(notifier=w353) -> (notifier out=w352:refnum<notifier>, current notification=w351:T10)  [unwired: 1 in, 3 out]
            n79 = Bundle By Name(cluster=w351, "Action"=w348) -> (w350:T10)
            n80 = Send Notification(notification=w350, notifier=w352) -> ()  [unwired: 1 in, 2 out]
          }
          event "Image Selection": Value Change {
            n81 = event-data() -> ("NewVal"=w362:i32)  [unwired: 1 in]
            n82 = Get Notifier Status(notifier=w370) -> (current notification=w368:T11[])  [unwired: 1 in, 4 out]
            n83 = Index Array(array=w368, index=w362) -> (element=w366:T11)
            n84 = Get Notifier Status(notifier=w369) -> (notifier out=w364:refnum<notifier>, current notification=w367:T10)  [unwired: 1 in, 3 out]
            n85 = Bundle By Name(cluster=w367, "Image Ref"=w366, "Action"=4Pi_Dual_DM_-_Mode_Scan_-_Scan_Actions."Exit") -> (w365:T10)
            n86 = Send Notification(notification=w365, notifier=w364) -> ()  [unwired: 1 in, 2 out]
          }
          event Value Change {
            n87 = event-data() -> ("NewVal"=w373:T4)  [unwired: 1 in]
            n88 = Get Notifier Status(notifier=w378) -> (notifier out=w375:refnum<notifier>, current notification=w377:T10)  [unwired: 1 in, 3 out]
            n89 = case shown="1" w373 {
              tunnel: [T24."Enabled" ("Disabled") T24."Disabled and Grayed Out" ("Disabled")] -> w372
              frame 0, Default {
              }
              frame 1 {
              }
            }
            n90 = Bundle By Name(cluster=w377, "Fit Type"=w373, "Action"=4Pi_Dual_DM_-_Mode_Scan_-_Scan_Actions."Exit") -> (w376:T10)
            n91 = Send Notification(notification=w376, notifier=w375) -> ()  [unwired: 1 in, 2 out]
            n92 = property on="Gaussian Initial Guesses" class="Clust (strict)"("DisabledEnum"=w372) -> ()  [unwired: 2 in, 2 out]
          }
          event Value Change {
            n93 = event-data() -> ("NewVal"=w384:T7)  [unwired: 1 in]
            n94 = Get Notifier Status(notifier=w386) -> (notifier out=w383:refnum<notifier>, current notification=w385:T10)  [unwired: 1 in, 3 out]
            n95 = Bundle By Name(cluster=w385, "Metric"=w384, "Action"=4Pi_Dual_DM_-_Mode_Scan_-_Scan_Actions."Exit") -> (w382:T10)
            n96 = Send Notification(notification=w382, notifier=w383) -> ()  [unwired: 1 in, 2 out]
          }
          event Value Change {
            n97 = event-data() -> ("NewVal"=w391:T3)  [unwired: 1 in]
            n98 = Get Notifier Status(notifier=w393) -> (notifier out=w390:refnum<notifier>, current notification=w392:T10)  [unwired: 1 in, 3 out]
            n99 = Bundle By Name(cluster=w392, "Image Type"=w391, "Action"=4Pi_Dual_DM_-_Mode_Scan_-_Scan_Actions."Exit") -> (w389:T10)
            n100 = Send Notification(notification=w389, notifier=w390) -> ()  [unwired: 1 in, 2 out]
          }
          event Value Change {
            n101 = event-data() -> ("NewVal"=w396:T5)  [unwired: 1 in]
            n102 = Get Notifier Status(notifier=w401) -> (notifier out=w398:refnum<notifier>, current notification=w400:T10)  [unwired: 1 in, 3 out]
            n103 = Bundle By Name(cluster=w400, "Gaussian Initial Guesses"=w396, "Action"=4Pi_Dual_DM_-_Mode_Scan_-_Scan_Actions."Exit") -> (w399:T10)
            n104 = Send Notification(notification=w399, notifier=w398) -> ()  [unwired: 1 in, 2 out]
          }
          event Value Change {
            n105 = event-data() -> ("NewVal"=w403:T6)  [unwired: 1 in]
            n106 = Get Notifier Status(notifier=w408) -> (notifier out=w405:refnum<notifier>, current notification=w407:T10)  [unwired: 1 in, 3 out]
            n107 = Bundle By Name(cluster=w407, "DM Scan Settings"=w403, "Action"=4Pi_Dual_DM_-_Mode_Scan_-_Scan_Actions."Exit") -> (w406:T10)
            n108 = Send Notification(notification=w406, notifier=w405) -> ()  [unwired: 1 in, 2 out]
          }
          event Value Change {
            n109 = event-data() -> ("NewVal"=w410:T8)  [unwired: 1 in]
            n110 = Get Notifier Status(notifier=w415) -> (notifier out=w412:refnum<notifier>, current notification=w414:T10)  [unwired: 1 in, 3 out]
            n111 = Bundle By Name(cluster=w414, "Threshold Mean Limits"=w410, "Action"=4Pi_Dual_DM_-_Mode_Scan_-_Scan_Actions."Exit") -> (w413:T10)
            n112 = Send Notification(notification=w413, notifier=w412) -> ()  [unwired: 1 in, 2 out]
          }
          event Value Change {
            n113 = event-data() -> ("NewVal"=w417:T1)  [unwired: 1 in]
            n114 = Get Notifier Status(notifier=w422) -> (notifier out=w419:refnum<notifier>, current notification=w421:T10)  [unwired: 1 in, 3 out]
            n115 = Bundle By Name(cluster=w421, "Blink Scan Settings"=w417, "Action"=4Pi_Dual_DM_-_Mode_Scan_-_Scan_Actions."Exit") -> (w420:T10)
            n116 = Send Notification(notification=w420, notifier=w419) -> ()  [unwired: 1 in, 2 out]
          }
          event "Exit": Value Change {
            n117 = event-data() -> ()  [unwired: 1 in, 1 out]
            n118 = Release Notifier(notifier=w429) -> ()  [unwired: 2 in, 3 out]
            n119 = Get Notifier Status(notifier=w427) -> (notifier out=w428:refnum<notifier>, current notification=w426:T10)  [unwired: 1 in, 3 out]
            n120 = Bundle By Name(cluster=w426, "Action"=4Pi_Dual_DM_-_Mode_Scan_-_Scan_Actions."Quit") -> (w425:T10)
            n121 = Send Notification(notification=w425, notifier=w428) -> ()  [unwired: 1 in, 2 out]
          }
        }
      }
      n122 = while {
        tunnel: w101 -> [w110]
        tunnel: w100 -> [w109]
        tunnel: w97 -> [w108]
        stop <- w104 stop-if-true
        n123 = Wait on Notification(notifier=w108, ignore previous (F)=TRUE) -> (notifier out=w105:refnum<notifier>, notification=w106:T10)  [unwired: 2 in, 2 out]
        n124 = Unbundle By Name(w106) -> ("Action"=w102:T9)
        n125 = Equal?(x=4Pi_Dual_DM_-_Mode_Scan_-_Scan_Actions."Quit" ("y"), y=w102) -> (x = y?=w104:bool)
        n126 = while {
          shift-right: [w118] -> _
          shift-left: w102 -> [w112]
          tunnel: w110 -> [w117]
          tunnel: w109 -> [w116]
          tunnel: w105 -> [w115]
          stop <- w119 stop-if-true
          n127 = Get Notifier Status(notifier=w115) -> (notifier out=w114:refnum<notifier>, current notification=w113:T10)  [unwired: 1 in, 3 out]
          n128 = case shown="\"Get Image\"" w112 {
            selector: w112 -> [_ _ _ _ _ _ _ _ w298]
            tunnel: [w120 w137 w161 w168 w203 w209 w272 w291 TRUE] -> w119
            tunnel: [4Pi_Dual_DM_-_Mode_Scan_-_Scan_Actions."Update Mode Amount" ("y") 4Pi_Dual_DM_-_Mode_Scan_-_Scan_Actions."Get Image" ("y") 4Pi_Dual_DM_-_Mode_Scan_-_Scan_Actions."Compute Metric" ("y") 4Pi_Dual_DM_-_Mode_Scan_-_Scan_Actions."Update Counter" ("y") w204 4Pi_Dual_DM_-_Mode_Scan_-_Scan_Actions."Apply Correction" ("y") 4Pi_Dual_DM_-_Mode_Scan_-_Scan_Actions."Exit" ("y") 4Pi_Dual_DM_-_Mode_Scan_-_Scan_Actions."Scan Mode" ("y") 4Pi_Dual_DM_-_Mode_Scan_-_Scan_Actions."Exit" ("y")] -> w118
            tunnel: w117 -> [_ w142 _ _ _ _ w275 _ w296]
            tunnel: w116 -> [_ w140 w167 _ _ _ _ _ _]
            tunnel: w114 -> [_ _ _ _ _ _ _ _ w297]
            tunnel: w113 -> [w123 w138 w165 w172 _ w212 _ _ _]
            tunnel: FALSE -> [w120 w137 w161 w168 w203 w209 w272 w291 _]
            frame "Scan Mode" {
              w127 = 4Pi_Dual_DM_-_Standard_Action."Read" ("Action")
              n129 = Unbundle By Name(w123) -> ("DM Scan Settings.Number of Steps"=w121:u16, "DM Scan Settings.Step Size (nm)"=w122:u16)
              n130 = call "4Pi Dual DM - Mirror Mode DUAL AE.vi"("Action"=w127) -> ("Mirror Modes Out"=w129:T25)  [unwired: 14 in]
              n131 = call "4Pi Dual DM - Active Mirror AE.vi"("Action"=w127) -> ("Active Mirror"=w128:i32)  [unwired: 14 in]
              n132 = Index Array(array=w129, index (col)=w128) -> (element=w126:cluster{"Mode":string, "Amplitude":dbl}[])  [unwired: 1 in]
              n133 = Initialize Array(0.0 ("element"), 0 ("dimension size")) -> (w130:dbl[])
              n134 = call "4Pi Dual DM - Mode Scan Data AE.vi"("Amplitude"=w130, "Action"=4Pi_Dual_DM_-_Standard_Action."Write", "Metric"=w130) -> ()  [unwired: 11 in, 2 out]
              n135 = Index Array(array=w126, index="Current Mode") -> (element=w135:cluster{"Mode":string, "Amplitude":dbl})
              n136 = Unbundle By Name(w135) -> ("Amplitude"=w136:dbl)
              n137 = call "4Pi Dual DM - Mode Scan Counter.vi"("Center Value"=w136, "Action"=4Pi_Dual_DM_-_Standard_Counter_Action."Initialize", "Mode"="Current Mode", "Number of Steps"=w121, "Step Size"=w122) -> ()  [unwired: 8 in, 3 out]
            }
            frame "Update Mode Amount" {
              n138 = flat-sequence {
                tunnel: w142 -> [w153]
                tunnel: [w153] -> w141
                tunnel: w141 -> [w156]
                tunnel: w140 -> [w160]
                tunnel: w138 -> [w159]
                frame #0 {
                  w149 = 4Pi_Dual_DM_-_Standard_Action."Read" ("Action")
                  n139 = call "4Pi Dual DM - Mirror Mode DUAL AE.vi"("Action"=w149) -> ("Mirror Modes Out"=w146:T25)  [unwired: 14 in]
                  n140 = call "4Pi Dual DM - Active Mirror AE.vi"("Action"=w149) -> ("Active Mirror"=w143:i32)  [unwired: 14 in]
                  n141 = Index Array(array=w146, index (col)=w143) -> (element=w148:cluster{"Mode":string, "Amplitude":dbl}[])  [unwired: 1 in]
                  n142 = call "4Pi Dual DM - Mode Scan Counter.vi"("Action"=4Pi_Dual_DM_-_Standard_Counter_Action."Get Count") -> ("Mode Amount"=w150:dbl, "Current Mode"=w151:i32)  [unwired: 12 in, 1 out]
                  n143 = Index Array(array=w148, index=w151) -> (element=w154:cluster{"Mode":string, "Amplitude":dbl})
                  n144 = Bundle By Name(cluster=w154, "Amplitude"=w150) -> (w155:cluster{"Mode":string, "Amplitude":dbl})
                  n145 = Replace Array Subset(array=w148, new element=w155, index=w151) -> (w144:cluster{"Mode":string, "Amplitude":dbl}[])
                  n146 = Replace Array Subset(array=w146, new element=w144, index (col)=w143) -> (w145:T25)  [unwired: 1 in]
                  n147 = call "4Pi Dual DM - Mirror Mode DUAL AE.vi"("Action"=4Pi_Dual_DM_-_Standard_Action."Write", "Mirror Modes In"=w145) -> ()  [unwired: 13 in, 1 out]
                }
                frame #1 {
                  n148 = Enqueue Element(queue=w156, element="Mirror Modes" ("name (unnamed)")) -> ()  [unwired: 2 in, 3 out]
                }
                frame #2 {
                  n149 = Unbundle By Name(w159) -> ("DM Scan Settings.Frame Delay"=w158:u32)
                  n150 = call "4Pi Dual DM - Confirm New Frame.vi"("Camera Notifier Name"=w160, "Wait No. (1)"=w158) -> ()  [unwired: 13 in, 1 out]
                }
              }
            }
            frame "Get Image" {
              n151 = Unbundle By Name(w165) -> ("Image Ref"=w164:T11, "DM Scan Settings.Frame Accumulations"=w162:u16)  [unwired: 1 out]
              n152 = call "4Pi Dual DM - Get Image.vi"("Camera Notifier Name"=w167, "Image Ref"=w164, "Frame Accums."=w162) -> ("Image Out"=→"Image":u16[][])  [unwired: 12 in]
            }
            frame "Compute Metric" {
              n153 = Unbundle By Name(w172) -> ("Metric"=w171:T7, "Threshold Mean Limits.Upper Limit"=w170:dbl, "Threshold Mean Limits.Lower Limit"=w169:dbl)
              n154 = property on="Image" class="IntGraph (strict)"() -> ("Value"=w175:u16[][])  [unwired: 2 in, 2 out]
              n155 = To Double Precision Float(number=w175) -> (double precision float=w174:dbl[][])
              n156 = case shown="1" w171 {
                tunnel: w174 -> [w189 w192 w197 w201]
                tunnel: [w187 w191 w195 w198] -> w181
                tunnel: w170 -> [_ _ w194 _]
                tunnel: w169 -> [_ _ w193 _]
                frame 0, Default {
                  n157 = Array Max & Min(array=w189) -> (max value=w188:dbl)  [unwired: 3 out]
                  n158 = To Double Precision Float(number=w188) -> (double precision float=w187:dbl)
                }
                frame 1 {
                  n159 = call "4Pi Dual DM - No Zeros Mean.vi"("Image IN"=w192, "STDev Factor"=0.0) -> ("No Zero Mean"=w191:dbl)  [unwired: 13 in]
                }
                frame 2 {
                  n160 = call "4Pi Dual DM - Threshold 2D Array.vi"("2D Array IN"=w197, "Upper Limit (Inclusive)"=w194, "Lower Limit (Inclusive)"=w193) -> ("Threshold Array Out"=w196:dbl[])  [unwired: 12 in]
                  n161 = call-poly <vilib>:"Mean.vi"("X"=w196) -> ("mean"=w195:dbl)  [unwired: 1 out]
                }
                frame 3 {
                  n162 = Array Size(array=w201) -> (size(s)=w202:i32[])
                  n163 = Multiply Array Elements(1:w202) -> (0:w200:i32)
                  n164 = Reshape Array(w201, w200) -> (w199:dbl[])
                  n165 = call-poly <vilib>:"Mean.vi"("X"=w199) -> ("mean"=w198:dbl)  [unwired: 1 out]
                }
              }
              n166 = call "4Pi Dual DM - Mode Scan Data AE.vi"("Action"=4Pi_Dual_DM_-_Standard_Action."Read") -> ("Amplitude Out"=w178:dbl[], "Metric Out"=w179:dbl[])  [unwired: 13 in]
              n167 = call "4Pi Dual DM - Mode Scan Counter.vi"("Action"=4Pi_Dual_DM_-_Standard_Counter_Action."Get Count") -> ("Mode Amount"=w180:dbl)  [unwired: 12 in, 2 out]
              n168 = Build Array (concatenate)(w179, w181) -> (w184:dbl[])
              n169 = Build Array (concatenate)(w178, w180) -> (w183:dbl[])
              n170 = call "4Pi Dual DM - Mode Scan Data AE.vi"("Amplitude"=w183, "Action"=4Pi_Dual_DM_-_Standard_Action."Write", "Metric"=w184) -> ()  [unwired: 11 in, 2 out]
              n171 = Bundle(w183, w184) -> (w185:cluster{dbl[], dbl[]})  [unwired: 1 in]
              n172 = Build Array(w185) -> (→"Metric":cluster{dbl[], dbl[]}[])
            }
            frame "Update Counter" {
              n173 = call "4Pi Dual DM - Mode Scan Counter.vi"("Action"=4Pi_Dual_DM_-_Standard_Counter_Action."Update Count") -> ("Scan Done?"=w207:bool)  [unwired: 12 in, 2 out]
              n174 = Select(t=4Pi_Dual_DM_-_Mode_Scan_-_Scan_Actions."Fit Data" ("y"), s=w207, f=4Pi_Dual_DM_-_Mode_Scan_-_Scan_Actions."Update Mode Amount" ("y")) -> (s? t:f=w204:T9)
            }
            frame "Fit Data" {
              n175 = Unbundle By Name(w212) -> ("Gaussian Initial Guesses"=w211:T5, "Fit Type"=w210:T4)
              n176 = call "4Pi Dual DM - Mode Scan Data AE.vi"("Action"=4Pi_Dual_DM_-_Standard_Action."Read") -> ("Amplitude Out"=w222:dbl[], "Metric Out"=w223:dbl[])  [unwired: 13 in]
              n177 = Bundle("Amplitude Out"=w222, "Metric Out"=w223) -> (w221:T26)  [unwired: 1 in]
              n178 = case shown="1" w210 {
                tunnel: w222 -> [w227 w271]
                tunnel: w223 -> [w255 w270]
                tunnel: [w246 w267] -> w216
                tunnel: [w245 w268] -> w219
                tunnel: [w244 w269] -> w218
                tunnel: w211 -> [w242 _]
                frame 0, Default {
                  n179 = To Double Precision Float(number=w255) -> (double precision float=w254:dbl[])
                  n180 = Array Max & Min(array=w227) -> (max value=w233:dbl, min value=w232:dbl)  [unwired: 2 out]
                  n181 = Unbundle By Name(w242) -> ("Amplitude"=w241:dbl, "Center Position"=w240:dbl, "Width (Sigma)"=w239:dbl, "Offset"=w238:dbl, "User Guesses"=w225:bool)
                  n182 = Array Max & Min(array=w254) -> (max value=w235:dbl, max index (indices)=w228:i32, min value=w234:dbl)  [unwired: 1 out]
                  n183 = Subtract(x=w233, y=w232) -> (x-y=w231:dbl)
                  n184 = Divide(x=w231, y=2.0) -> (x/y=w229:dbl)
                  n185 = Bundle By Name(cluster=T21 {"initial amplitude"=nan, "initial center"=nan, "initial standard deviation"=nan, "offset"=nan} ("initial guess"), "initial amplitude"=w241, "initial center"=w240, "initial standard deviation"=w239, "offset"=w238) -> (w236:T21)
                  n186 = Index Array(array=w227, index=w228) -> (element=w226:dbl)
                  n187 = Bundle(w235, "Numeric"=w226, w229, w234) -> (w253:cluster{dbl, "Numeric":dbl, dbl, dbl})  [unwired: 1 in]
                  n188 = Select(t=w236, s=w225, f=w253) -> (s? t:f=w237:T27)
                  n189 = call <vilib>:"Gaussian Peak Fit.vi"("Y"=w254, "initial guess"=w237, "X"=w227, "parameter bounds"=T22 {"amp min"=0.0, "amp max"=100000.0, "center min"=-100.0, "center max"=100.0, "deviation min"=0.0, "deviation max"=1000.0, "offset min"=0.0, "offset max"=1000.0}) -> ("offset"=w249:dbl, "amplitude"=w251:dbl, "center"=w246:dbl, "standard deviation"=w250:dbl)  [unwired: 5 in, 3 out]
                  n190 = Build Array(w251, w246, w250, w249) -> (w248:dbl[])
                  n191 = call "4Pi Dual DM - 1D Gaussian.vi"("Parameters In"=w248, "Number of Points"=1000.0, "Max X Value"=w233, "Min X Value"=w232) -> ("X Values"=w245:dbl[], "Y Values"=w244:dbl[])  [unwired: 10 in]
                }
                frame 1 {
                  w265 = T28 2 items=["Least Square", "Least Absolute Residual", "Bisquare"] ("method")
                  # "LV often can't find this file. It should be located at C:\\Program Files\\National Instruments\\LabVIEW 2016\\examples\\Mathematics\\Fitting\\support"
                  n192 = To Double Precision Float(number=w270) -> (double precision float=w266:dbl[])
                  n193 = call <vilib>:"General Polynomial Fit.vi"("Y"=w266, "polynomial order"=2, "X"=w271, "method"=w265) -> ("Polynomial Coefficients"=w262:dbl[])  [unwired: 8 in, 3 out]
                  n194 = Array Max & Min(array=w271) -> (max value=w258:dbl, min value=w257:dbl)  [unwired: 2 out]
                  n195 = call "Regression Equation String.vi"("coefficients"=w262, "precision"=3, "fit type"=T23."Polynomial") -> ("Formula"=w260:string)  [unwired: 8 in]
                  n196 = call <vilib>:"Eval y=f(x) Optimal Step.vi"("number of points"=u32 3000, "formula"=w260, "end"=w258, "start"=w257) -> ("Y Values"=w269:dbl[], "X Values"=w268:dbl[])  [unwired: 1 in, 2 out]
                  n197 = Array Max & Min(array=w269) -> (max index (indices)=w256:i32)  [unwired: 3 out]
                  n198 = Index Array(array=w268, index=w256) -> (element=w267:dbl)
                }
              }
              n199 = Bundle("X Values"=w219, "Y Values"=w218) -> (w217:cluster{"X Values":dbl[], "Y Values":dbl[]})  [unwired: 1 in]
              n200 = Build Array(w221, w217) -> (w220:cluster{"X Values":dbl[], "Y Values":dbl[]}[])
              n201 = property on="Metric" class="XYGraph (strict)"("Cursor.Cursor X"=w216, "Cursor.Cursor Y"=-10000.0 ("Cursor.Cursor Position:Cursor X"), "Cursor.Visible"=TRUE, "Value"=w220) -> ()  [unwired: 2 in, 2 out]
            }
            frame "Apply Correction" {
              n202 = flat-sequence {
                tunnel: w275 -> [w288]
                tunnel: [w288] -> w274
                tunnel: w274 -> [w289]
                frame #0 {
                  w280 = 4Pi_Dual_DM_-_Standard_Action."Read" ("Action")
                  n203 = call "4Pi Dual DM - Mirror Mode DUAL AE.vi"("Action"=w280) -> ("Mirror Modes Out"=w283:T25)  [unwired: 14 in]
                  n204 = call "4Pi Dual DM - Active Mirror AE.vi"("Action"=w280) -> ("Active Mirror"=w286:i32)  [unwired: 14 in]
                  n205 = property on="Metric" class="XYGraph (strict)"() -> ("Cursor.Cursor X"=w287:dbl)  [unwired: 2 in, 2 out]
                  n206 = Index Array(array=w283, index (col)=w286) -> (element=w281:cluster{"Mode":string, "Amplitude":dbl}[])  [unwired: 1 in]
                  n207 = call "4Pi Dual DM - Mode Scan Counter.vi"("Action"=4Pi_Dual_DM_-_Standard_Counter_Action."Get Count") -> ("Current Mode"=w279:i32)  [unwired: 12 in, 2 out]
                  n208 = Index Array(array=w281, index=w279) -> (element=w277:cluster{"Mode":string, "Amplitude":dbl})
                  n209 = Bundle By Name(cluster=w277, "Amplitude"=w287) -> (w276:cluster{"Mode":string, "Amplitude":dbl})
                  n210 = Replace Array Subset(array=w281, new element=w276, index=w279) -> (w285:cluster{"Mode":string, "Amplitude":dbl}[])
                  n211 = Replace Array Subset(array=w283, new element=w285, index (col)=w286) -> (w284:T25)  [unwired: 1 in]
                  n212 = call "4Pi Dual DM - Mirror Mode DUAL AE.vi"("Action"=4Pi_Dual_DM_-_Standard_Action."Write", "Mirror Modes In"=w284) -> ()  [unwired: 13 in, 1 out]
                }
                frame #1 {
                  n213 = Enqueue Element(queue=w289, element="Mirror Modes" ("name (unnamed)")) -> ()  [unwired: 2 in, 3 out]
                }
              }
            }
            frame "Scan Next Mode" {
              n214 = call "4Pi Dual DM - Mode Scan Counter.vi"("Action"=4Pi_Dual_DM_-_Standard_Counter_Action."Get Count") -> ("Current Mode"=w294:i32)  [unwired: 12 in, 2 out]
              n215 = Increment(x=w294) -> (x+1=w295:i32)
              n216 = local write "Current Mode"(w295) -> ()
            }
            frame "Exit", "Quit" {
              n217 = case shown="\"Quit\"" w298 {
                tunnel: w297 -> [w319 _]
                tunnel: w296 -> [w320 _]
                frame "Quit" {
                  w317 = T12 {"Image Ref Index"=0, "Image Type"=0, "Fit Type"=0, "Metric"=1, "DM Scan Settings"={"Frame Delay"=1, "Frame Accumulations"=2, "Number of Steps"=8, "Step Size (nm)"=80}, "Threshold Mean Limits"={"Upper Limit"=10000.0, "Lower Limit"=0.0}, "Gaussian Initial Guesses"={"Amplitude"=2500.0, "Center Position"=0.0, "Width (Sigma)"=200.0, "Offset"=500.0, "User Guesses"=TRUE}, "Blink Scan Settings"={"Blink Analysis Type"=1, "Blink ROI Box Width"=0, "Blink Threshold"=0.0}}  # Last Used Scan Settings
                  n218 = Release Notifier(notifier=w319, force destroy? (F)=TRUE) -> (last notification=w318:T10)  [unwired: 1 in, 2 out]
                  n219 = Release Queue(queue=w320) -> ()  [unwired: 2 in, 3 out]
                  n220 = Unbundle By Name(w318) -> ("Image Type"=w316:T3, "Fit Type"=w314:T4, "Metric"=w313:T7, "DM Scan Settings"=w312:T6, "Threshold Mean Limits"=w311:T8, "Gaussian Initial Guesses"=w310:T5, "Blink Scan Settings"=w309:T1)
                  n221 = local read "Image Selection"() -> (w315:i32)
                  n222 = control-ref of="This VI"() -> (w308:refnum<vi>)
                  n223 = property class="VI"(reference=w308) -> ("Path"=w307:path)  [unwired: 1 in, 2 out]
                  n224 = Bundle By Name(cluster=w317, "Image Ref Index"=w315, "Image Type"=w316, "Fit Type"=w314, "Metric"=w313, "DM Scan Settings"=w312, "Threshold Mean Limits"=w311, "Gaussian Initial Guesses"=w310, "Blink Scan Settings"=w309) -> (w303:T12)
                  n225 = Strip Path(path=w307) -> (stripped path=w306:path)  [unwired: 1 out]
                  n226 = Strip Path(path=w306) -> (stripped path=w305:path)  [unwired: 1 out]
                  n227 = Build Path(base path=w305, name or relative path="4Pi Dual DM - Default Files\\Last Used Scan Settings.json") -> (appended path=w301:path)
                  n228 = Flatten To JSON(anything=w303) -> (JSON string=w302:string)  [unwired: 2 in, 1 out]
                  n229 = Write to Text File(file (use dialog)=w301, text=w302) -> ()  [unwired: 2 in, 3 out]
                }
                frame "Exit", Default {
                }
              }
            }
          }
        }
      }
    }
    frame Error {
    }
  }
